vi "1DTurnMain.vi"() -> ()   [LabVIEW 2017]
panel:
  in  "Target A?":bool
  in  "Target B":dbl
  out "Encoder Distance":cluster{"Output":dbl, "dx/dt":dbl}(graph)={"Output"=3.552713678800501e-14, "dx/dt"=0.819812390525771}
  in  "Config":T1={"Gear Reduction"=8.7, "Wheel Radius (m)"=0.076, "# Motors"=3, "coeff of friction"=0.1, "Mass (kg)"=55.0, "Motor"={"Ke (V)"=0.0183, "R (ohms)"=0.14, "KT (Nm/A)"=0.0183, "Tf (Nm)"=0.015}}
  in  "Gains":T2={"Gains"={"FFV"=0.0055, "FFA"=0.0025, "Vel PID"={"P"=0.05, "I"=0.0, "D"=0.0}}, "Pos PID"={"P"=0.05, "I"=0.0, "D"=0.0}, "MinVoltage"=0.05, "Effective Trackwidth"=30.0, "Effective Trackwidth CCW"=30.0} {"Pos PID"."D" format="%.3f"; "Pos PID"."I" format="%.3f"; "Pos PID"."P" format="%.3f"; "Gains"."Vel PID"."D" format="%.3f"; "Gains"."Vel PID"."I" format="%.3f"; "Gains"."Vel PID"."P" format="%.3f"}
  out "Power":dbl(graph)
  in  "StartAngle":dbl
  out "Done?":bool=TRUE
  out "Vel":cluster{"Output":dbl, "dx/dt":dbl}(graph)={"Output"=0.0, "dx/dt"=0.35426442870059566}
  out "Angle":cluster{"Distance":dbl, "CurrentAngle":dbl}(graph)={"Distance"=0.0, "CurrentAngle"=3.131452664643774}
  in  "Target A":dbl
  in  "MaxVel":dbl=80.0
  in  "MaxAccel":dbl=100.0
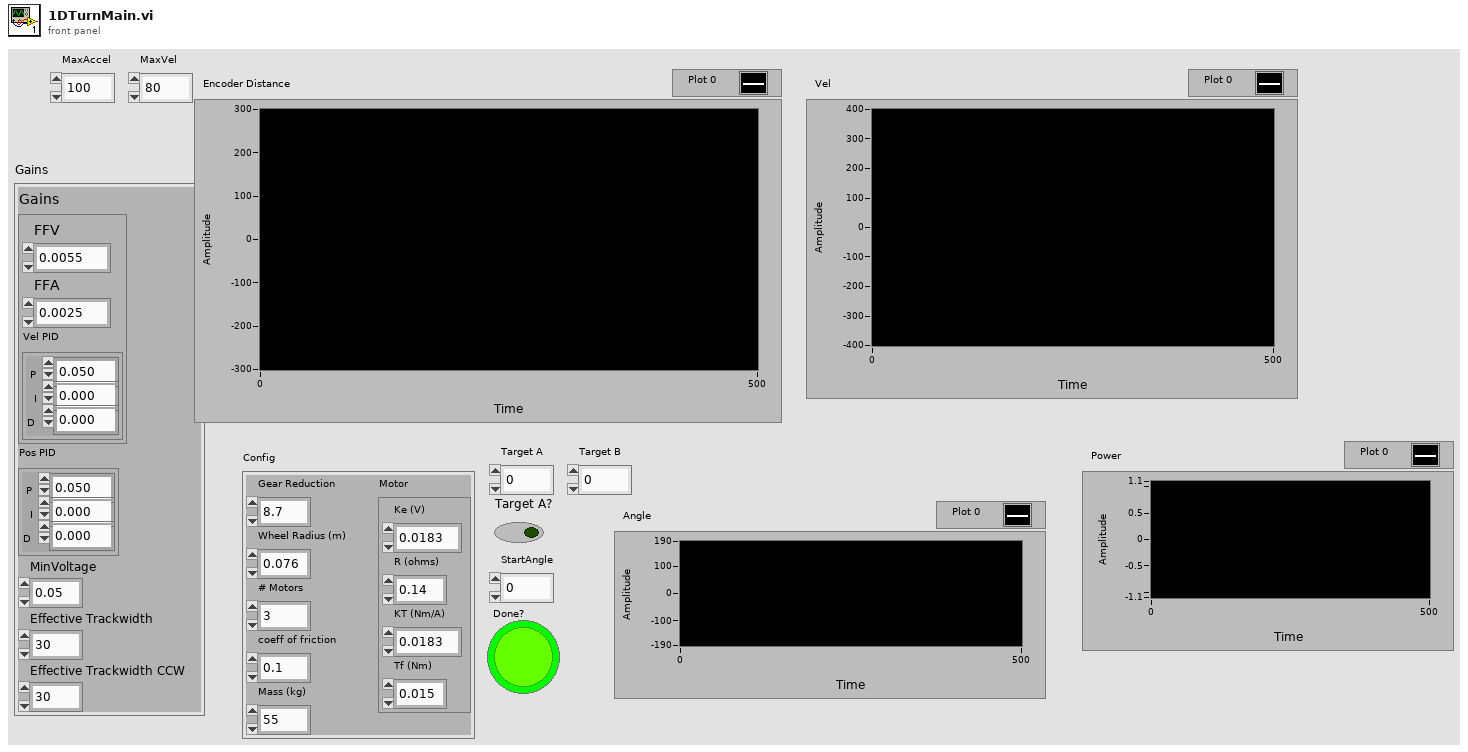
[diagram p1: front panel]
types:
  T1 = cluster{"Gear Reduction":dbl, "Wheel Radius (m)":dbl, "# Motors":u32, "coeff of friction":dbl, "Mass (kg)":dbl, "Motor":cluster{"Ke (V)":dbl, "R (ohms)":dbl, "KT (Nm/A)":dbl, "Tf (Nm)":dbl}}
  T2 = cluster{"Gains":cluster{"FFV":dbl, "FFA":dbl, "Vel PID":cluster{"P":dbl, "I":dbl, "D":dbl}}, "Pos PID":cluster{"P":dbl, "I":dbl, "D":dbl}, "MinVoltage":dbl, "Effective Trackwidth":dbl, "Effective Trackwidth CCW":dbl}
  T3 = cluster{"angle":dbl, "angular vel":dbl, "Left Distance":dbl, "Left vel":dbl, "Right Distance":dbl, "Right vel":dbl}
  T4 = cluster{dbl, "dx/dt":dbl, "Left Distance":dbl, "dx/dt":dbl, "Right Distance":dbl, "dx/dt":dbl}
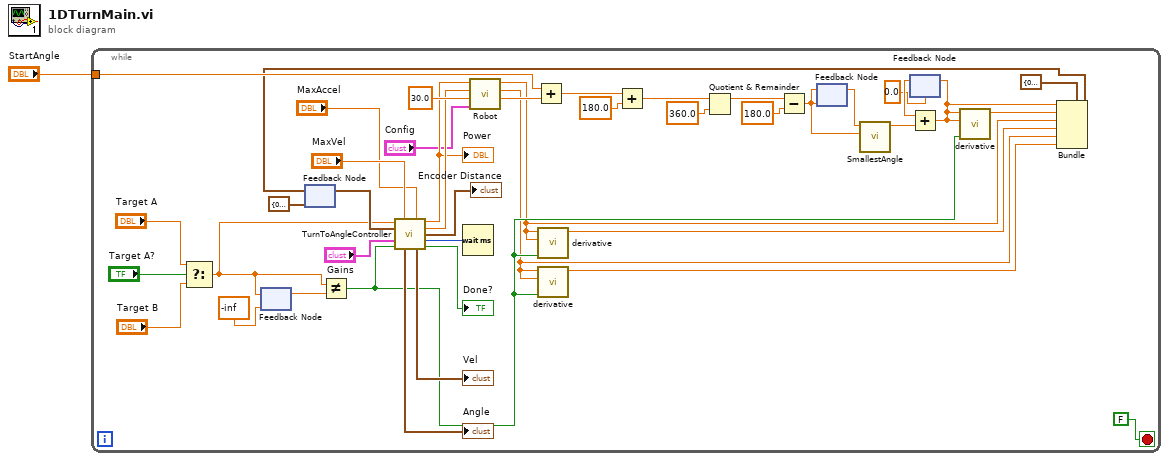
[diagram p0: block diagram]
diagram:
  n1 = while {
    tunnel: "StartAngle" -> [w26]
    stop <- FALSE stop-if-true
    n2 = Select(t="Target A", s="Target A?", f="Target B") -> (s? t:f=w2:dbl)
    n3 = feedback-in #1(w2) -> ()
    n4 = feedback #1(-inf ("TargetAngle")) -> (w34:dbl)
    n5 = feedback #2(T4 {0.0, "dx/dt"=0.0, "Left Distance"=0.0, "dx/dt"=0.0, "Right Distance"=0.0, "dx/dt"=0.0}) -> (w13:T4)
    n6 = Not Equal?(x=w2, y=w34) -> (x != y?=w21:bool)
    n7 = call "TurnToAngleController.vi"("TargetAngle"=w2, "MaxVel"="MaxVel", "MaxAccel"="MaxAccel", "Robot"=w13, "Gains"="Gains", "Reset"=w21) -> ("LeftPower"=w10:dbl, "RightPower"=w38:dbl, "Encoder Distance"=→"Encoder Distance":cluster{"Output":dbl, "dx/dt":dbl}, "Delay"=w42:u32, "Angle"=→"Angle":cluster{"Distance":dbl, "CurrentAngle":dbl}, "VelGraph"=→"Vel":cluster{"Output":dbl, "dx/dt":dbl}, "Done"=→"Done?":bool)  [unwired: 3 in]
    "Power" <- w10
    n8 = Wait (ms)(milliseconds to wait=w42) -> ()  [unwired: 1 out]
    n9 = call "Robot.vi"("Config"="Config", "WheelBase"=30.0, "Right Value"=w38, "Left Value"=w10) -> ("Angle"=w28:dbl, "Right Distance"=w16:dbl, "Left Distance"=w18:dbl)  [unwired: 5 in]
    n10 = Add(x=w26, y=w28) -> (x+y=w27:dbl)
    n11 = call "derivative.vi"("Reset"=w21, "Starting value"=w18, "x"=w18) -> ("dx/dt"=w17:dbl)  [unwired: 8 in]
    n12 = call "derivative.vi"("Reset"=w21, "Starting value"=w16, "x"=w16) -> ("dx/dt"=w15:dbl)  [unwired: 8 in]
    n13 = Add(x=w27, y=180.0) -> (x+y=w32:dbl)
    n14 = Quotient & Remainder(x=w32, y=360.0) -> (x-y*floor(x/y)=w30:dbl)  [unwired: 1 out]
    n15 = Subtract(x=w30, y=180.0) -> (x-y=w22:dbl)
    n16 = feedback #3(w22) -> (w23:dbl)
    n17 = feedback-in #3(w22) -> ()
    n18 = call "SmallestAngle.vi"("Angle B"=w22, "Angle A"=w23) -> ("Smallest A to B"=w24:dbl)  [unwired: 9 in]
    n19 = feedback #4(0.0) -> (w25:dbl)
    n20 = Add(x=w25, y=w24) -> (x+y=w20:dbl)
    n21 = feedback-in #4(w20) -> ()
    n22 = call "derivative.vi"("Reset"=w21, "Starting value"=w20, "x"=w20) -> ("dx/dt"=w19:dbl)  [unwired: 8 in]
    n23 = Bundle(cluster=T3 {"angle"=0.0, "angular vel"=0.0, "Left Distance"=0.0, "Left vel"=0.0, "Right Distance"=0.0, "Right vel"=0.0} ("Robot"), "angle"=w20, "angular vel"=w19, "Left Distance"=w18, "Left vel"=w17, "Right Distance"=w16, "Right vel"=w15) -> (w14:T3)
    n24 = feedback-in #2(w14) -> ()
  }
